vi "task2.vi"() -> ()   [LabVIEW 2020]
panel:
  out "countTotal":i64
  out "Average iterations":dbl
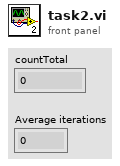
[diagram p1: front panel]
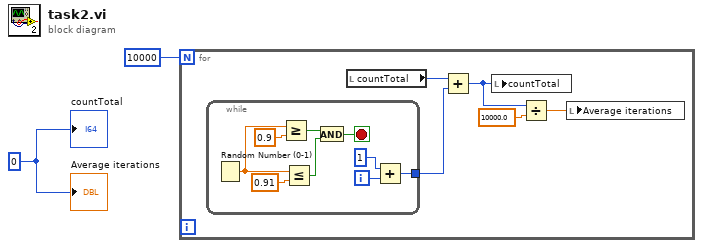
[diagram p0: block diagram]
diagram:
  w1 = i64 0 ("countall")
  n1 = for {
    N: 10000 -> [_]
    n2 = while {
      tunnel: [w8] -> w7
      i -> [w11]
      stop <- w10 stop-if-true
      n3 = Random Number (0-1)() -> (number: 0 to 1=w9:dbl)
      n4 = Greater Or Equal?(x=w9, y=0.9) -> (x >= y?=w16:bool)
      n5 = Less Or Equal?(x=w9, y=0.91) -> (x <= y?=w13:bool)
      n6 = And(x=w16, y=w13) -> (x .and. y?=w10:bool)
      n7 = Add(x=1, y=w11) -> (x+y=w8:i32)
    }
    n8 = local read "countTotal"() -> (w6:i64)
    n9 = Add(x=w6, y=w7) -> (x+y=w3:i64)
    n10 = local write "countTotal"(w3) -> ()
    n11 = Divide(x=w3, y=10000.0) -> (x/y=w5:dbl)
    n12 = local write "Average iterations"(w5) -> ()
  }
  "countTotal" <- w1
  "Average iterations" <- w1
